vi "peirce_calcErrorFunction.vi"(1 "x":dbl format="%#_13g") -> (0 "PhiX":dbl)   [LabVIEW 2016]
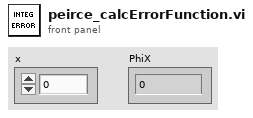
[diagram p1: front panel]
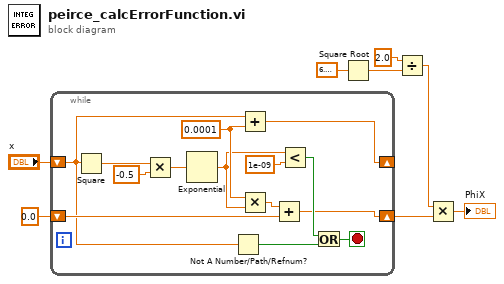
[diagram p0: block diagram]
diagram:
  n1 = while {
    shift-right: [w19] -> _
    shift-left: "x" -> [w11]
    shift-right: [w12] -> w2
    shift-left: 0.0 -> [w16]
    stop <- w10 stop-if-true
    w18 = 0.0001 ("y")
    n2 = Square(x=w11) -> (x^2=w22:dbl)
    n3 = Multiply(x=w22, y=-0.5) -> (x*y=w20:dbl)
    n4 = Exponential(1:w20) -> (0:w15:dbl)
    n5 = Not A Number/Path/Refnum?(number/path/refnum=w11) -> (NaN/Path/Refnum?=w9:bool)
    n6 = Add(x=w11, y=w18) -> (x+y=w19:dbl)
    n7 = Multiply(x=w18, y=w15) -> (x*y=w17:dbl)
    n8 = Add(x=w17, y=w16) -> (x+y=w12:dbl)
    n9 = Less?(x=w15, y=1e-09) -> (x < y?=w13:bool)
    n10 = Or(x=w13, y=w9) -> (x .or. y?=w10:bool)
  }
  n11 = Square Root(x=6.283185307179586) -> (sqrt(x)=w4:dbl)
  n12 = Divide(x=2.0, y=w4) -> (x/y=w7:dbl)
  n13 = Multiply(x=w7, y=w2) -> (x*y=→"PhiX":dbl)
